vi "Keyboard.vi"(7 "Array":u32[](array[numeric])) -> (8 "step":dbl)   [LabVIEW 2010]
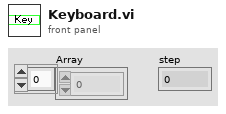
[diagram p1: front panel]
types:
  T1 = enum16{"0", "1", "2", "3", "4", "5", "6", "7", "8", "9", "A", "B", "C", "D", "E", "F", "G", "H", "I", "J", "K", "L", "M", "N", "O", "P", "Q", "R", "S", "T", "U", "V", "W", "X", "Y", "Z", "F1", "F2", "F3", "F4", "F5", "F6", "F7", "F8", "F9", "F10", "F11", "F12", "F13", "F14", "F15", "ADD", "BACK", "BACKSLASH", "CAPITAL", "COMMA", "DECIMAL", "DELETE", "DIVIDE", "DOWN", "END", "EQUALS", "ESCAPE", "GRAVE (`)", "HOME", "INSERT", "LBRACKET", "LCONTROL", "LEFT", "L ALT", "LSHIFT", "LWIN", "MINUS", "MULTIPLY", "NEXT", "NUMLOCK", "NUMPAD_0", "NUMPAD_1", "NUMPAD_2", "NUMPAD_3", "NUMPAD_4", "NUMPAD_5", "NUMPAD_6", "NUMPAD_7", "NUMPAD_8", "NUMPAD_9", "PAUSE", "PERIOD", "PRIOR (PG UP)", "RBRACKET", "RCONTROL", "RETURN", "RIGHT", "R ALT", "RSHIFT", "RWIN", "SCROLL", "SEMICOLON", "SLASH", "SPACE", "SUBTRACT", "TAB", "UP", "ENTER (num pad)", "' (quote)"}
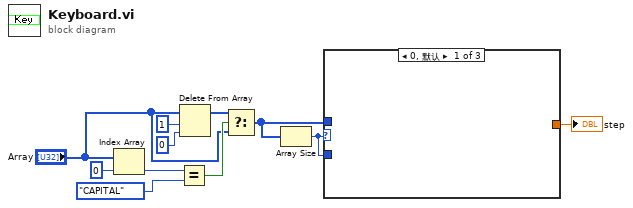
[diagram p0: block diagram]
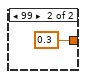
[diagram p3: hidden frame]
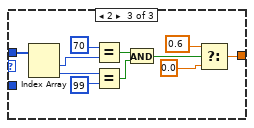
[diagram p4: hidden frame]
diagram:
  n1 = Index Array(array="Array", index=0) -> (element=w8:u32)
  n2 = Equal?(x=w8, y=T1."CAPITAL" ("keyType 3")) -> (x = y?=w7:bool)
  n3 = Delete From Array(array="Array", length=1, index=0) -> (array with subset deleted=w4:u32[])  [unwired: 1 out]
  n4 = Select(t=w4, s=w7, f="Array") -> (s? t:f=w2:u32[])
  n5 = Array Size(array=w2) -> (size(s)=w10:i32)
  n6 = case shown="0, 默认" w10 {
    tunnel: w10 -> [_ w14 _]
    tunnel: w2 -> [_ w13 w28]
    tunnel: [_ w12 w23] -> w11
    frame 0, Default {
    }
    frame 1 {
      n7 = for {
        N: w14 -> [_]
        tunnel: w13 -> [w16] mode=indexing
        tunnel: [w15] -> w12
        n8 = case shown="0, 默认" w16 {
          tunnel: [_ 0.3] -> w15
          frame 0, Default {
          }
          frame 99 {
          }
        }
      }
    }
    frame 2 {
      n9 = Index Array(array=w28) -> (element #1=w27:u32, element #2=w26:u32)  [unwired: 2 in]
      n10 = Equal?(x=u32 70, y=w27) -> (x = y?=w25:bool)
      n11 = Equal?(x=w26, y=u32 99) -> (x = y?=w24:bool)
      n12 = And(x=w25, y=w24) -> (x .and. y?=w22:bool)
      n13 = Select(t=0.6, s=w22, f=0.0) -> (s? t:f=w23:dbl)
    }
  }
  "step" <- w11
